vi "StringWithNoOfSpace.vi"(9 "StringLength":i32, 11 "String":string) -> (2 "OutString":string)   [LabVIEW 2012]
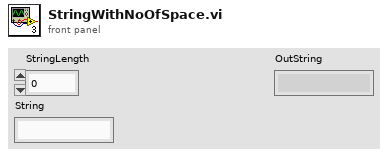
[diagram p1: front panel]
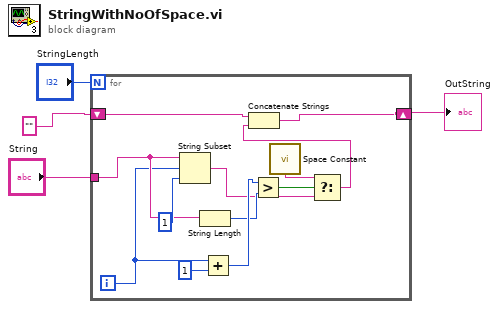
[diagram p0: block diagram]
diagram:
  n1 = for {
    N: "StringLength" -> [_]
    tunnel: "String" -> [w13]
    shift-right: [w14] -> w1
    shift-left: "" ("string") -> [w15]
    i -> [w12]
    n2 = String Subset(string=w13, offset (0)=w12, length (rest)=1 ("length (rest)")) -> (substring=w7:string)
    n3 = String Length(string=w13) -> (length=w9:i32)
    n4 = Add(x=w12, y=1) -> (x+y=w10:i32)
    n5 = Greater?(x=w10, y=w9) -> (0:w8:bool)
    n6 = call <vilib>:"Space Constant.vi"() -> ("String"=w5:string)
    n7 = Select(t=w5, s=w8, f=w7) -> (s? t:f=w6:string)
    n8 = Concatenate Strings(w15, w6) -> (w14:string)
  }
  "OutString" <- w1
